vi "Write Node Array.vi"(8 "error in":errorcluster, 10 "Node Array":refnum<class "Node.lvclass">[](array[class]), 11 "XML Document in":refnum<class "XML Document.lvclass">) -> (0 "error out":errorcluster, 3 "XML Document out":refnum<class "XML Document.lvclass">)   [LabVIEW 2014, in "XML Document.lvclass"]
uses:
  XML Document.lvclass
  Node_class/Node.lvclass
  XML Document.lvclass/XML Document.ctl
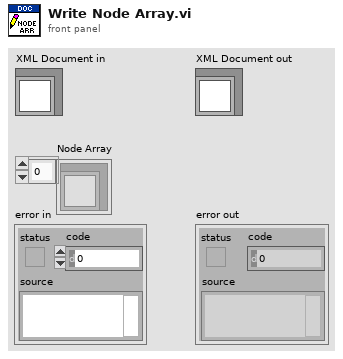
[diagram p1: front panel]
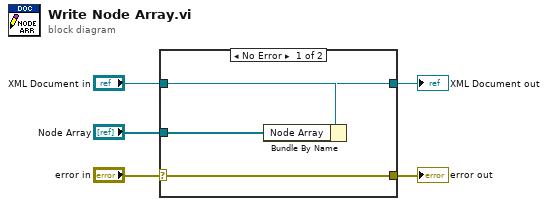
[diagram p0: block diagram]
diagram:
  n1 = case shown="No Error" "error in" {
    selector: "error in" -> [w9 w10]
    tunnel: [w9 w10] -> w4
    tunnel: [w7 w11] -> w2
    tunnel: "XML Document in" -> [w8 w11]
    tunnel: "Node Array" -> [w6 _]
    frame No Error {
      n2 = Bundle By Name(cluster=w8, "Node Array"=w6) -> (w7:refnum<class "XML Document.lvclass">)
    }
    frame Error {
    }
  }
  "error out" <- w4
  "XML Document out" <- w2
